vi "Calcula_CRC.vi"(4 "Message Data":u8[](array[numeric]) format="%.0x") -> (0 "Calculated CRC":u16 format="%.0x", 1 "String":string)   [LabVIEW 2017]
panel:
  out "Send message":u8[](array[numeric]) format="%.0x"
  out "CRC HB":u8 format="%.0x"
  out "CRC LB":u8 format="%.0x"
  in  "Increment":u16=1
  out "Message Length":u16
  # "Bytes + 2"
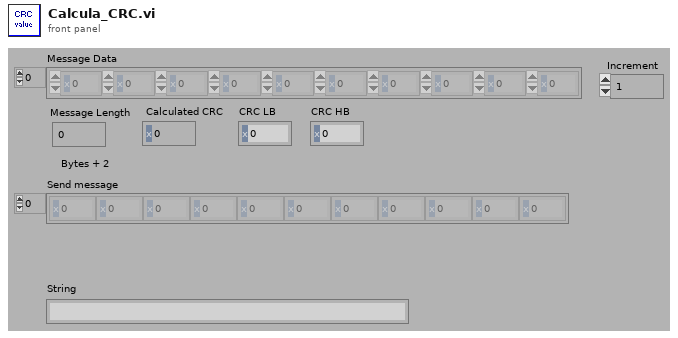
[diagram p1: front panel]
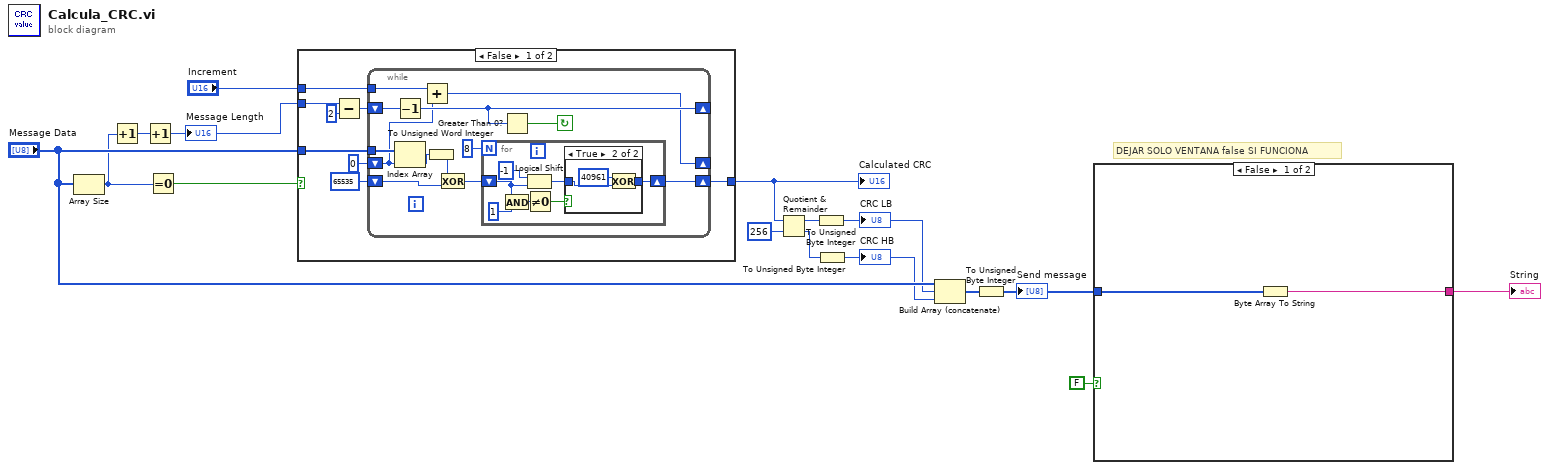
[diagram p0: block diagram]
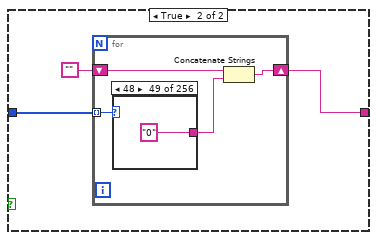
[diagram p2: hidden frame]
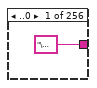
[diagram p3: hidden frame]
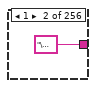
[diagram p4: hidden frame]
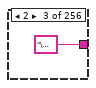
[diagram p5: hidden frame]
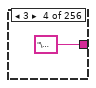
[diagram p6: hidden frame]
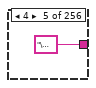
[diagram p7: hidden frame]
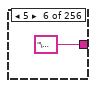
[diagram p8: hidden frame]
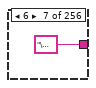
[diagram p9: hidden frame]
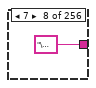
[diagram p10: hidden frame]
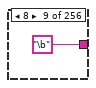
[diagram p11: hidden frame]
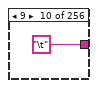
[diagram p12: hidden frame]
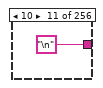
[diagram p13: hidden frame]
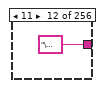
[diagram p14: hidden frame]
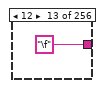
[diagram p15: hidden frame]
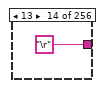
[diagram p16: hidden frame]
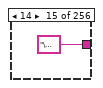
[diagram p17: hidden frame]
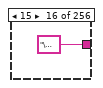
[diagram p18: hidden frame]
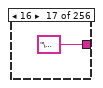
[diagram p19: hidden frame]
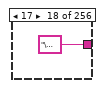
[diagram p20: hidden frame]
diagram:
  # "DEJAR SOLO VENTANA false SI FUNCIONA"
  n1 = Array Size(array="Message Data") -> (size(s)=w9:i32)
  n2 = Increment(x=w9) -> (x+1=w11:i32)
  n3 = Increment(x=w11) -> (x+1=w10:i32)
  "Message Length" <- w10
  n4 = Equal To 0?(x=w9) -> (x = 0?=w15:bool)
  n5 = case shown="False" w15 {
    tunnel: "Message Data" -> [w24 _]
    tunnel: [w23 u16 65535] -> w14
    tunnel: "Increment" -> [w22 _]
    tunnel: w10 -> [w18 _]
    frame False {
      n6 = Subtract(x=w18, y=u16 2) -> (x-y=w17:i32)
      n7 = while {
        tunnel: w22 -> [w31]
        shift-left: u16 65535 -> [w33]
        shift-right: [w25] -> w23
        tunnel: w24 -> [w34]
        shift-left: u16 0 -> [w30]
        shift-right: [w29] -> _
        shift-left: w17 -> [w37]
        shift-right: [w36] -> _
        stop <- w35 continue-if-true
        n8 = Decrement(x=w37) -> (x-1=w36:i32)
        n9 = Index Array(array=w34, index=w30) -> (element=w28:u8)
        n10 = Add(x=w31, y=w30) -> (x+y=w29:u16)
        n11 = To Unsigned Word Integer(number=w28) -> (unsigned 16bit integer=w27:u16)
        n12 = Exclusive Or(1:w33, 2:w27) -> (0:w26:u16)
        n13 = for {
          N: 8 -> [_]
          shift-right: [w38] -> w25
          shift-left: w26 -> [w39]
          n14 = And(x=w39, y=u16 1) -> (x .and. y?=w41:u16)
          n15 = Logical Shift(y=-1, x=w39) -> (x << y=w40:u16)
          n16 = Not Equal To 0?(x=w41) -> (x != 0?=w42:bool)
          n17 = case shown="True" w42 {
            tunnel: [w45 w46] -> w38
            tunnel: w40 -> [w45 w47]
            frame False {
            }
            frame True {
              n18 = Exclusive Or(1:w47, 2:u16 40961) -> (0:w46:u16)
            }
          }
        }
        n19 = Greater Than 0?(x=w36) -> (x > 0?=w35:bool)
      }
    }
    frame True {
    }
  }
  "Calculated CRC" <- w14
  n20 = Quotient & Remainder(x=w14, y=u16 256) -> (x-y*floor(x/y)=w3:u16, floor(x/y)=w4:u16)
  n21 = To Unsigned Byte Integer(number=w3) -> (unsigned 8bit integer=w2:u8)
  "CRC LB" <- w2
  n22 = To Unsigned Byte Integer(number=w4) -> (unsigned 8bit integer=w1:u8)
  "CRC HB" <- w1
  n23 = Build Array (concatenate)("Message Data", w2, w1) -> (w6:u8[])
  n24 = To Unsigned Byte Integer(number=w6) -> (unsigned 8bit integer=w5:u8[])
  "Send message" <- w5
  n25 = case shown="False" FALSE {
    tunnel: w5 -> [w51 w54]
    tunnel: [w50 w52] -> w8
    frame False {
      n26 = Byte Array To String(unsigned byte array=w51) -> (string=w50:string)
    }
    frame True {
      n27 = for {
        tunnel: w54 -> [w56] mode=indexing
        shift-right: [w58] -> w52
        shift-left: "" -> [w57]
        n28 = case shown="48" w56 {
          tunnel: ["\u0000" "\u0001" "\u0002" "\u0003" "\u0004" "\u0005" "\u0006" "\u0007" "\b" "\t" "\n" "\u000b" "\f" "\r" "\u000e" "\u000f" "\u0010" "\u0011" "\u0012" "\u0013" "\u0014" "\u0015" "\u0016" "\u0017" "\u0018" "\u0019" "\u001a" "\u001b" "\u001c" "\u001d" "\u001e" "\u001f" " " "!" "\"" "#" "$" "%" "&" "'" "(" ")" "*" "+" "," "-" "." "/" "0" "1" "2" "3" "4" "5" "6" "7" "8" "9" ":" ";" "<" "=" ">" "?" "@" "A" "B" "C" "D" "E" "F" "G" "H" "I" "J" "K" "L" "M" "N" "O" "P" "Q" "R" "S" "T" "U" "V" "W" "X" "Y" "Z" "[" "\\" "]" "^" "_" "`" "a" "b" "c" "d" "e" "f" "g" "h" "i" "j" "k" "l" "m" "n" "o" "p" "q" "r" "s" "t" "u" "v" "w" "x" "y" "z" "{" "|" "}" "~" "" "€" "" "‚" "ƒ" "„" "…" "†" "‡" "ˆ" "‰" "Š" "‹" "Œ" "" "Ž" "" "" "‘" "’" "“" "”" "•" "–" "—" "˜" "™" "š" "›" "œ" "" "ž" "Ÿ" " " "¡" "¢" "£" "¤" "¥" "¦" "§" "¨" "©" "ª" "«" "¬" "­" "®" "¯" "°" "±" "²" "³" "´" "µ" "¶" "·" "¸" "¹" "º" "»" "¼" "½" "¾" "¿" "À" "Á" "Â" "Ã" "Ä" "Å" "Æ" "Ç" "È" "É" "Ê" "Ë" "Ì" "Í" "Î" "Ï" "Ð" "Ñ" "Ò" "Ó" "Ô" "Õ" "Ö" "×" "Ø" "Ù" "Ú" "Û" "Ü" "Ý" "Þ" "ß" "à" "á" "â" "ã" "ä" "å" "æ" "ç" "è" "é" "ê" "ë" "ì" "í" "î" "ï" "ð" "ñ" "ò" "ó" "ô" "õ" "ö" "÷" "ø" "ù" "ú" "û" "ü" "ý" "þ" "ÿ"] -> w55
          frame ..0 {
          }
          frame 1 {
          }
          frame 2 {
          }
          frame 3 {
          }
          frame 4 {
          }
          frame 5 {
          }
          frame 6 {
          }
          frame 7 {
          }
          frame 8 {
          }
          frame 9 {
          }
          frame 10 {
          }
          frame 11 {
          }
          frame 12 {
          }
          frame 13 {
          }
          frame 14 {
          }
          frame 15 {
          }
          frame 16 {
          }
          frame 17 {
          }
          frame 18 {
          }
          frame 19 {
          }
          frame 20 {
          }
          frame 21 {
          }
          frame 22 {
          }
          frame 23 {
          }
          frame 24 {
          }
          frame 25 {
          }
          frame 26 {
          }
          frame 27 {
          }
          frame 28 {
          }
          frame 29 {
          }
          frame 30 {
          }
          frame 31 {
          }
          frame 32 {
          }
          frame 33 {
          }
          frame 34 {
          }
          frame 35 {
          }
          frame 36 {
          }
          frame 37 {
          }
          frame 38 {
          }
          frame 39 {
          }
          frame 40 {
          }
          frame 41 {
          }
          frame 42 {
          }
          frame 43 {
          }
          frame 44 {
          }
          frame 45 {
          }
          frame 46 {
          }
          frame 47 {
          }
          frame 48 {
          }
          frame 49 {
          }
          frame 50 {
          }
          frame 51 {
          }
          frame 52 {
          }
          frame 53 {
          }
          frame 54 {
          }
          frame 55 {
          }
          frame 56 {
          }
          frame 57 {
          }
          frame 58 {
          }
          frame 59 {
          }
          frame 60 {
          }
          frame 61 {
          }
          frame 62 {
          }
          frame 63 {
          }
          frame 64 {
          }
          frame 65 {
          }
          frame 66 {
          }
          frame 67 {
          }
          frame 68 {
          }
          frame 69 {
          }
          frame 70 {
          }
          frame 71 {
          }
          frame 72 {
          }
          frame 73 {
          }
          frame 74 {
          }
          frame 75 {
          }
          frame 76 {
          }
          frame 77 {
          }
          frame 78 {
          }
          frame 79 {
          }
          frame 80 {
          }
          frame 81 {
          }
          frame 82 {
          }
          frame 83 {
          }
          frame 84 {
          }
          frame 85 {
          }
          frame 86 {
          }
          frame 87 {
          }
          frame 88 {
          }
          frame 89 {
          }
          frame 90 {
          }
          frame 91 {
          }
          frame 92 {
          }
          frame 93 {
          }
          frame 94 {
          }
          frame 95 {
          }
          frame 96 {
          }
          frame 97 {
          }
          frame 98 {
          }
          frame 99 {
          }
          frame 100 {
          }
          frame 101 {
          }
          frame 102 {
          }
          frame 103 {
          }
          frame 104 {
          }
          frame 105 {
          }
          frame 106 {
          }
          frame 107 {
          }
          frame 108 {
          }
          frame 109 {
          }
          frame 110 {
          }
          frame 111 {
          }
          frame 112 {
          }
          frame 113 {
          }
          frame 114 {
          }
          frame 115 {
          }
          frame 116 {
          }
          frame 117 {
          }
          frame 118 {
          }
          frame 119 {
          }
          frame 120 {
          }
          frame 121 {
          }
          frame 122 {
          }
          frame 123 {
          }
          frame 124 {
          }
          frame 125 {
          }
          frame 126 {
          }
          frame 127 {
          }
          frame 128 {
          }
          frame 129 {
          }
          frame 130 {
          }
          frame 131 {
          }
          frame 132 {
          }
          frame 133 {
          }
          frame 134 {
          }
          frame 135 {
          }
          frame 136 {
          }
          frame 137 {
          }
          frame 138 {
          }
          frame 139 {
          }
          frame 140 {
          }
          frame 141 {
          }
          frame 142 {
          }
          frame 143 {
          }
          frame 144 {
          }
          frame 145 {
          }
          frame 146 {
          }
          frame 147 {
          }
          frame 148 {
          }
          frame 149 {
          }
          frame 150 {
          }
          frame 151 {
          }
          frame 152 {
          }
          frame 153 {
          }
          frame 154 {
          }
          frame 155 {
          }
          frame 156 {
          }
          frame 157 {
          }
          frame 158 {
          }
          frame 159 {
          }
          frame 160 {
          }
          frame 161 {
          }
          frame 162 {
          }
          frame 163 {
          }
          frame 164 {
          }
          frame 165 {
          }
          frame 166 {
          }
          frame 167 {
          }
          frame 168 {
          }
          frame 169 {
          }
          frame 170 {
          }
          frame 171 {
          }
          frame 172 {
          }
          frame 173 {
          }
          frame 174 {
          }
          frame 175 {
          }
          frame 176 {
          }
          frame 177 {
          }
          frame 178 {
          }
          frame 179 {
          }
          frame 180 {
          }
          frame 181 {
          }
          frame 182 {
          }
          frame 183 {
          }
          frame 184 {
          }
          frame 185 {
          }
          frame 186 {
          }
          frame 187 {
          }
          frame 188 {
          }
          frame 189 {
          }
          frame 190 {
          }
          frame 191 {
          }
          frame 192 {
          }
          frame 193 {
          }
          frame 194 {
          }
          frame 195 {
          }
          frame 196 {
          }
          frame 197 {
          }
          frame 198 {
          }
          frame 199 {
          }
          frame 200 {
          }
          frame 201 {
          }
          frame 202 {
          }
          frame 203 {
          }
          frame 204 {
          }
          frame 205 {
          }
          frame 206 {
          }
          frame 207 {
          }
          frame 208 {
          }
          frame 209 {
          }
          frame 210 {
          }
          frame 211 {
          }
          frame 212 {
          }
          frame 213 {
          }
          frame 214 {
          }
          frame 215 {
          }
          frame 216 {
          }
          frame 217 {
          }
          frame 218 {
          }
          frame 219 {
          }
          frame 220 {
          }
          frame 221 {
          }
          frame 222 {
          }
          frame 223 {
          }
          frame 224 {
          }
          frame 225 {
          }
          frame 226 {
          }
          frame 227 {
          }
          frame 228 {
          }
          frame 229 {
          }
          frame 230 {
          }
          frame 231 {
          }
          frame 232 {
          }
          frame 233 {
          }
          frame 234 {
          }
          frame 235 {
          }
          frame 236 {
          }
          frame 237 {
          }
          frame 238 {
          }
          frame 239 {
          }
          frame 240 {
          }
          frame 241 {
          }
          frame 242 {
          }
          frame 243 {
          }
          frame 244 {
          }
          frame 245 {
          }
          frame 246 {
          }
          frame 247 {
          }
          frame 248 {
          }
          frame 249 {
          }
          frame 250 {
          }
          frame 251 {
          }
          frame 252 {
          }
          frame 253 {
          }
          frame 254 {
          }
          frame 255.. {
          }
        }
        n29 = Concatenate Strings(w57, w55) -> (w58:string)
      }
    }
  }
  "String" <- w8
